vi "IMAQdx_getAttribute_Bool.vi"(3 "error in (no error)":errorcluster, 4 "Attribute Name":string, 5 "IMAQdx Session":T1) -> (0 "error out":errorcluster, 1 "IMAQdx Attribute":variant, 2 "dup IMAQdx Session":T1)   [LabVIEW 2014, in "HGF_VisionTools.lvlib"]
doc: "This VI reads IMAQdx attribute value of type boolean and its properties. Value is returned as Variant and properties as Variant attributes."
uses:
  HGF_VisionTools.lvlib
  <resource>/objmgr/imaqdx.rc
  <vilib>/userdefined/High Color/IMAQdx.ctl
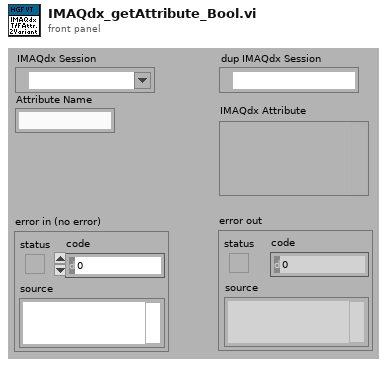
[diagram p1: front panel]
types:
  T1 = typedef "IMAQdx.ctl" = refnum<k21>
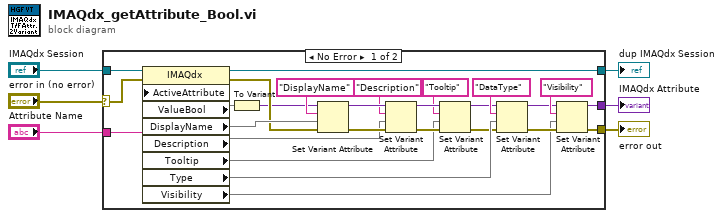
[diagram p0: block diagram]
diagram:
  n1 = case shown="No Error" "error in (no error)" {
    selector: "error in (no error)" -> [w7 w34]
    tunnel: "IMAQdx Session" -> [w33 w35]
    tunnel: "Attribute Name" -> [w32 _]
    tunnel: [w31 w35] -> w4
    tunnel: [w11 _] -> w3
    tunnel: [w10 w34] -> w2
    frame No Error {
      n2 = property class="IMAQdx"(reference=w33, error in=w7, "ActiveAttribute"=w32) -> (reference out=w31:T1, error out=w28:errorcluster, "ValueBool"=w27, "DisplayName"=w29, "Description"=w18, "Tooltip"=w17, "Type"=w16, "Visibility"=w12)
      n3 = To Variant(anything=w27) -> (Variant=w26:variant)
      n4 = Set Variant Attribute(Variant=w26, name="DisplayName", value=w29, error in=w28) -> (Variant out=w25:variant, error out=w22:errorcluster)  [unwired: 1 out]
      n5 = Set Variant Attribute(Variant=w25, name="Description", value=w18, error in=w22) -> (Variant out=w24:variant, error out=w23:errorcluster)  [unwired: 1 out]
      n6 = Set Variant Attribute(Variant=w24, name="Tooltip", value=w17, error in=w23) -> (Variant out=w9:variant, error out=w8:errorcluster)  [unwired: 1 out]
      n7 = Set Variant Attribute(Variant=w9, name="DataType", value=w16, error in=w8) -> (Variant out=w13:variant, error out=w14:errorcluster)  [unwired: 1 out]
      n8 = Set Variant Attribute(Variant=w13, name="Visibility", value=w12, error in=w14) -> (Variant out=w11:variant, error out=w10:errorcluster)  [unwired: 1 out]
    }
    frame Error {
    }
  }
  "IMAQdx Attribute" <- w3
  "dup IMAQdx Session" <- w4
  "error out" <- w2
